vi "Main_real.vi"() -> ()   [LabVIEW 2023]
panel:
  in  "On/Off":bool
  out "On/Off Light":bool
  in  "Exit":bool
  out "Data Chart":dbl(graph)
  in  "Sample time [s]":dbl=10.0
  in  "Sensor Type":string(combo)
  in  "AddSensor Button":bool
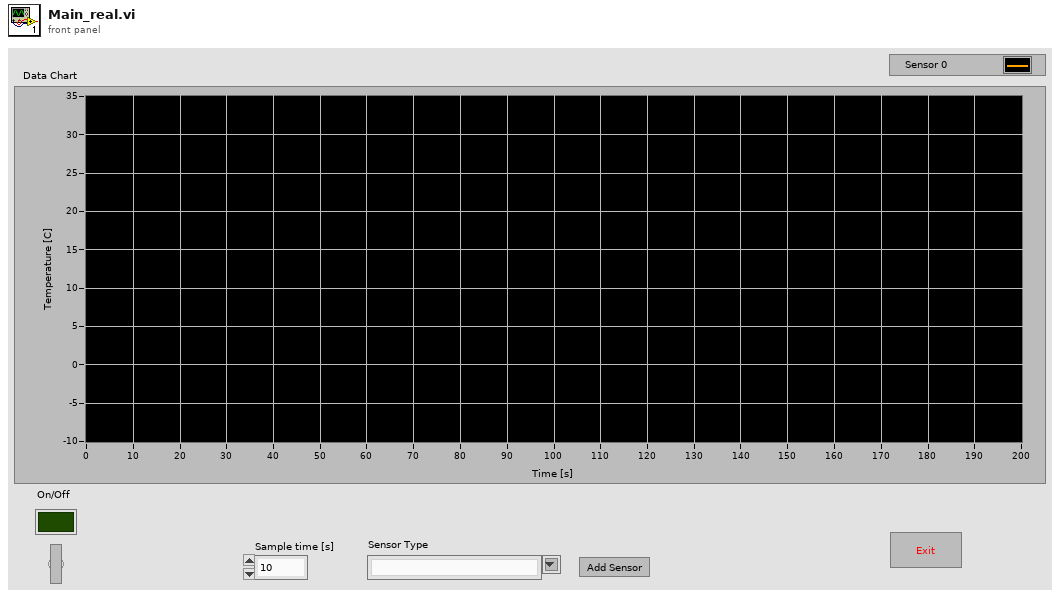
[diagram p1: front panel]
types:
  T1 = typedef "NI_Database_API.lvlib/Conn ObjectReference.ctl" = refnum<k1>
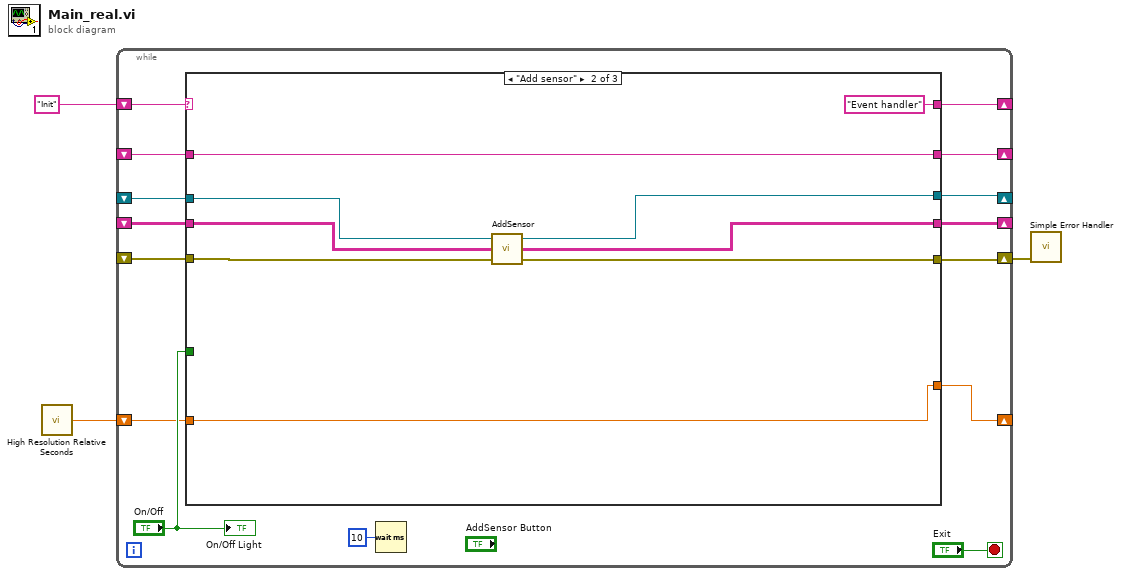
[diagram p0: block diagram]
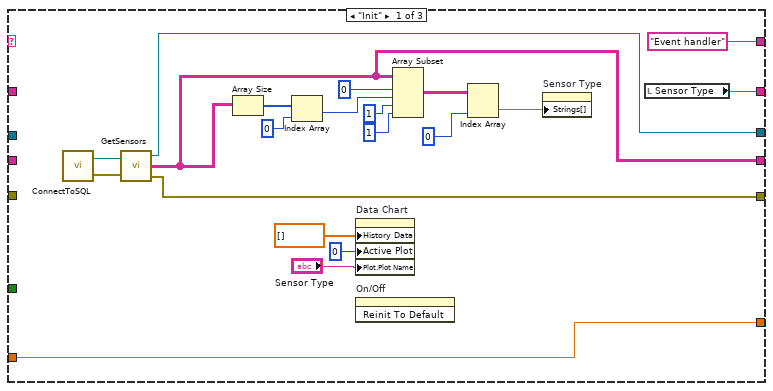
[diagram p2: hidden frame]
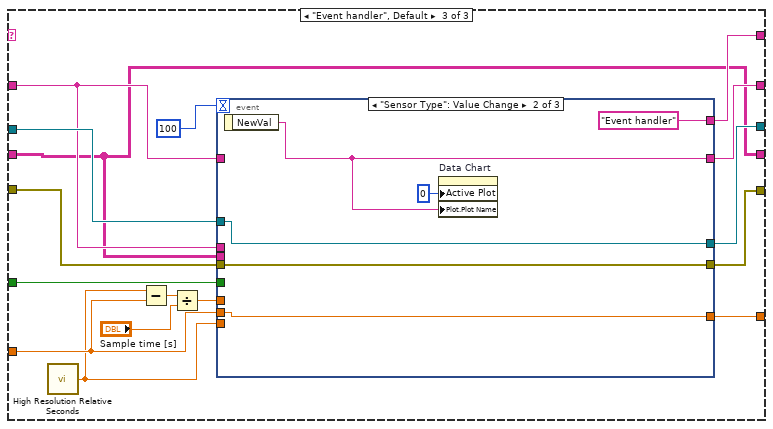
[diagram p3: hidden frame]
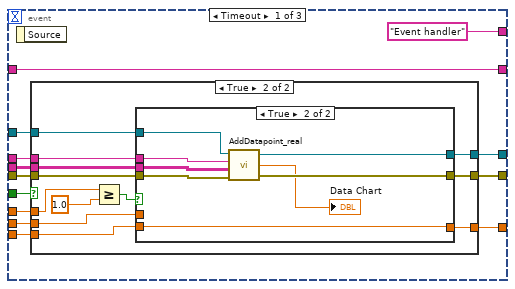
[diagram p4: hidden frame]
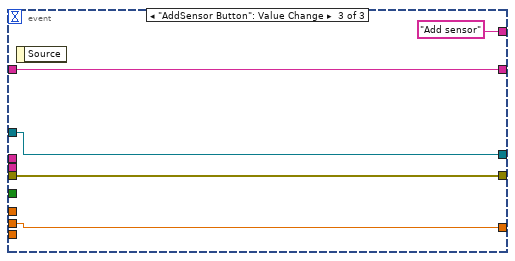
[diagram p7: hidden frame]
diagram:
  n1 = call <vilib>:"High Resolution Relative Seconds.vi"() -> ("relative seconds"=w1:dbl)
  n2 = while {
    shift-right: [w10] -> _
    shift-left: _ -> [w16]
    shift-right: [w15] -> _
    shift-left: "Init" -> [w17]
    shift-right: [w14] -> _
    shift-left: _ -> [w11]
    shift-right: [w13] -> w2
    shift-left: _ -> [w12]
    shift-right: [w7] -> _
    shift-left: w1 -> [w6]
    shift-right: [w5] -> _
    shift-left: _ -> [w4]
    stop <- "Exit" stop-if-true
    n3 = case shown="\"Add sensor\"" w17 {
      tunnel: [w33 w43 w57] -> w13
      tunnel: w16 -> [_ w41 w50]
      tunnel: ["Event handler" "Event handler" w62] -> w15
      tunnel: [w31 w42 w58] -> w14
      tunnel: w12 -> [_ w45 w59]
      tunnel: w11 -> [_ w47 w60]
      tunnel: [w23 w41 w49] -> w10
      tunnel: "On/Off" -> [_ _ w61]
      tunnel: [w37 w44 w54] -> w7
      tunnel: w6 -> [w37 w44 w53]
      tunnel: [w22 w39 w48] -> w5
      tunnel: w4 -> [_ w40 w48]
      frame "Init" {
        n4 = call "ConnectToSQL.vi"() -> ("error out"=w34:errorcluster, "connection reference"=w35:T1)  [unwired: 2 in]
        n5 = call "GetSensors.vi"("connection reference"=w35, "error in (no error)"=w34) -> ("connection reference 2"=w31:T1, "data"=w22:string[][], "error out"=w33:errorcluster)
        n6 = Array Size(array=w22) -> (size(s)=w28:i32[])
        n7 = Index Array(array=w28, index=0) -> (element=w26:i32)
        n8 = property on="Data Chart" class="WFChart (strict)"("History Data"=dbl[] [], "Active Plot"=u32 0, "Plot.Plot Name"="Sensor Type") -> ()  [unwired: 2 in, 2 out]
        n9 = invoke on="On/Off" class="Bool (strict)" method="Reinit To Default"() -> ()  [unwired: 3 in, 3 out]
        n10 = Array Subset(array=w22, index (row)=0 ("index"), length (row)=w26, index (col)=1 ("index"), length (col)=1 ("length")) -> (w21:string[][])
        n11 = Index Array(array=w21, index (col)=0 ("dimension size")) -> (element=w24:string[])  [unwired: 1 in]
        n12 = property on="Sensor Type" class="CmbBox"("Strings[]"=w24) -> ()  [unwired: 2 in, 2 out]
        n13 = local read "Sensor Type"() -> (w23:string)
      }
      frame "Add sensor" {
        n14 = call "AddSensor.vi"("error in (no error)"=w45, "Sensors in"=w40, "connection reference in"=w47) -> ("error out"=w43:errorcluster, "Sensors out"=w39:string[][], "connection reference out"=w42:T1)
      }
      frame "Event handler", Default {
        n15 = call <vilib>:"High Resolution Relative Seconds.vi"() -> ("relative seconds"=w52:dbl)
        n16 = Subtract(x=w52, y=w53) -> (x-y=w56:dbl)
        n17 = Divide(x=w56, y="Sample time [s]") -> (x/y=w55:dbl)
        n18 = event shown="[1] \"Sensor Type\": Value Change" {
          selector: _ -> [_ _ _]
          dyn-events: _ -> [_ _ _]
          timeout: 100 -> [_ _ _]
          tunnel: ["Event handler" "Event handler" "Add sensor"] -> w62
          tunnel: w61 -> [w75 _ _]
          tunnel: w60 -> [w74 w108 w111]
          tunnel: w59 -> [w73 w107 w112]
          tunnel: [w72 w108 w111] -> w58
          tunnel: [w71 w107 w112] -> w57
          tunnel: w50 -> [w70 _ _]
          tunnel: w55 -> [w69 _ _]
          tunnel: [w68 w105 w113] -> w54
          tunnel: w53 -> [w67 w105 w113]
          tunnel: w52 -> [w66 _ _]
          tunnel: [w65 w104 w109] -> w49
          tunnel: w50 -> [w65 _ w109]
          tunnel: w48 -> [w64 _ _]
          event Timeout {
            n19 = event-data() -> ()  [unwired: 1 in, 1 out]
            n20 = case shown="True" w75 {
              tunnel: w74 -> [w79 w91]
              tunnel: w73 -> [w78 w90]
              tunnel: [w79 w89] -> w72
              tunnel: [w78 w88] -> w71
              tunnel: w70 -> [_ w87]
              tunnel: w69 -> [_ w84]
              tunnel: [w77 w86] -> w68
              tunnel: w67 -> [w77 w85]
              tunnel: w66 -> [_ w81]
              tunnel: w64 -> [_ w80]
              frame False {
              }
              frame True {
                n21 = Greater Or Equal?(x=w84, y=1.0) -> (x >= y?=w83:bool)
                n22 = case shown="True" w83 {
                  tunnel: w91 -> [w93 w102]
                  tunnel: w90 -> [w92 w101]
                  tunnel: [w93 w100] -> w89
                  tunnel: [w92 w99] -> w88
                  tunnel: w87 -> [_ w96]
                  tunnel: [w94 w98] -> w86
                  tunnel: w85 -> [w94 _]
                  tunnel: w81 -> [_ w98]
                  tunnel: w80 -> [_ w95]
                  frame False {
                  }
                  frame True {
                    n23 = call "AddDatapoint_real.vi"("error in (no error)"=w101, "Sensor info"=w95, "Sensor Type"=w96, "connection reference in"=w102) -> ("error out"=w99:errorcluster, "Temperature"=→"Data Chart":dbl, "connection reference out"=w100:T1)
                  }
                }
              }
            }
          }
          event "Sensor Type": Value Change {
            n24 = event-data() -> ("NewVal"=w104:string)  [unwired: 1 in]
            n25 = property on="Data Chart" class="WFChart (strict)"("Active Plot"=u32 0, "Plot.Plot Name"=w104) -> ()  [unwired: 2 in, 2 out]
          }
          event "AddSensor Button": Value Change {
            n26 = event-data() -> ()  [unwired: 1 in, 1 out]
          }
        }
      }
    }
    n27 = Wait (ms)(milliseconds to wait=u32 10) -> ()  [unwired: 1 out]
    "On/Off Light" <- "On/Off"
  }
  n28 = call <vilib>:"Simple Error Handler.vi"("error in (no error)"=w2) -> ()  [unwired: 4 in, 5 out]
